vi "AM.vi"() -> ()   [LabVIEW 2017]
uses:
  <vilib>/sound2/lvsound2.llb/Sampling Mode.ctl
  <vilib>/sound2/lvsound2.llb/Sound Data Format.ctl
  <vilib>/Utility/error.llb/DialogType.ctl
  <vilib>/express/express analysis/Spectral/Block/exnSpectralBlock spectral measurements RMS poly.vi
  <vilib>/express/express analysis/Spectral/Block/exnSpectralBlock spectral measurements RMS WFM.vi
  <vilib>/sound2/lvsound2.llb/Sound Output Write (DBL Single).vi
  <vilib>/express/express analysis/Spectral/XNode/ExpressSpectralMeasurementsBlockNode.xnode
panel:
  in  "stop":bool
  out "Ausgang: Zeitbild":dbl[](graph)
  out "Ausgang: Frequenzbild":cluster{"f0":dbl, "df":dbl, "magnitude":dbl[]}(graph)={"f0"=0.0, "df"=2.2675736961451248e-05, "magnitude"=array[22050 elements]}
  in  "Modulationsgrad m":dbl=0.2
  in  "Signalamplitude 2":dbl=3.0
  in  "Signalamplitude 1":dbl=1.0
  in  "Signalfrequenz 2":dbl=1000.0
  in  "Signalfrequenz 1":dbl=700.0
  in  "Trägerfrequenz":dbl=10000.0
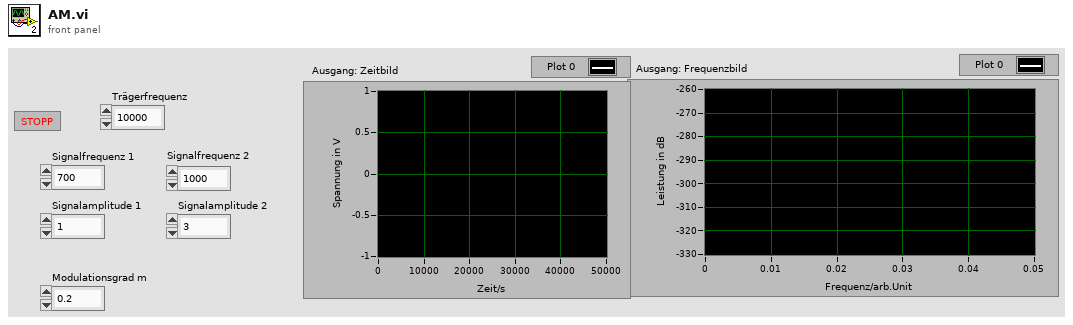
[diagram p1: front panel]
types:
  T1 = typedef "Sound Data Format.ctl" = cluster{"sample rate (S/s)":dbl, "number of channels":i32, "bits per sample":i32}
  T2 = cluster{"averaging mode":u16, "weighting mode":u16, "number of averages":u32}
  T3 = cluster{"dB On (F)":bool, "unwrap phase (F)":bool, "convert to degree (F)":bool}
  T4 = typedef "DialogType.ctl" = u16
  T5 = typedef "Sampling Mode.ctl" = i32
  T6 = typedef "Sound Output Task ID.ctl" = u32
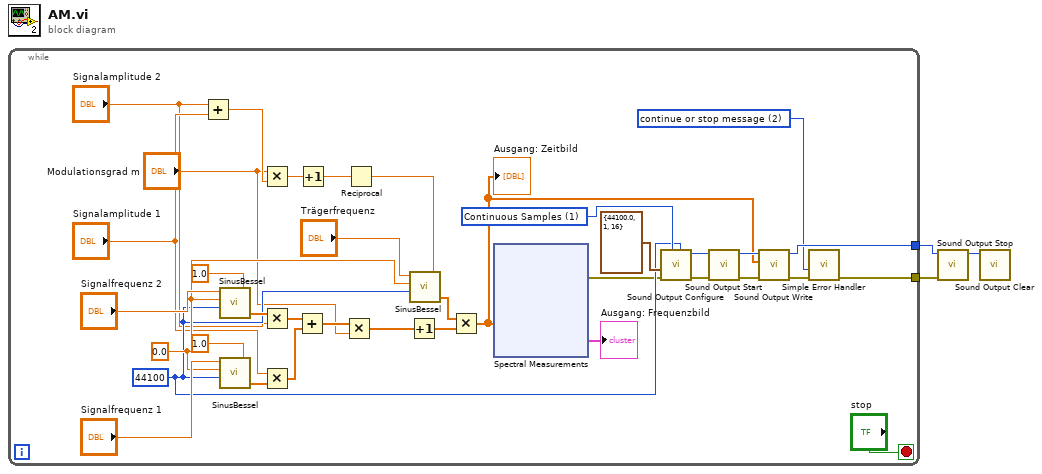
[diagram p0: block diagram]
diagram:
  n1 = while {
    tunnel: [w15] -> w2
    tunnel: [w17] -> w1
    stop <- "stop" stop-if-true
    w14 = T4 2 items=["no dialog", "OK message", "continue or stop message", "OK message + warnings", "continue/stop + warnings"] ("type of dialog (OK msg:1)")
    w13 = 44100 ("number of samples/ch")
    w24 = T5 1 items=["Finite Samples", "Continuous Samples"] ("sample mode")
    w33 = 0.0 ("Phase phi")
    n2 = Add(x="Signalamplitude 2", y="Signalamplitude 1") -> (x+y=w9:dbl)
    n3 = call "SinusBessel.vi"("Amplitude A"=1.0, "Zahl der Punkte N"=w13, "Phase phi"=w33, "Frequenz f"="Signalfrequenz 2") -> ("y"=w37:dbl[])  [unwired: 1 in, 1 out]
    n4 = call "SinusBessel.vi"("Amplitude A"=1.0, "Zahl der Punkte N"=w13, "Phase phi"=w33, "Frequenz f"="Signalfrequenz 1") -> ("y"=w29:dbl[])  [unwired: 1 in, 1 out]
    n5 = Multiply(x="Modulationsgrad m", y=w9) -> (x*y=w7:dbl)
    n6 = Multiply(x=w37, y="Signalamplitude 2") -> (x*y=w25:dbl[])
    n7 = Multiply(x="Signalamplitude 1", y=w29) -> (x*y=w27:dbl[])
    n8 = Add(x=w25, y=w27) -> (x+y=w36:dbl[])
    n9 = Increment(x=w7) -> (x+1=w6:dbl)
    n10 = Multiply(x=w36, y="Modulationsgrad m") -> (x*y=w35:dbl[])
    n11 = Reciprocal(x=w6) -> (1/x=w5:dbl)
    n12 = Increment(x=w35) -> (x+1=w32:dbl[])
    n13 = call "SinusBessel.vi"("Amplitude A"=w5, "Zahl der Punkte N"=w13, "Phase phi"=w33, "Frequenz f"="Trägerfrequenz") -> ("y"=w31:dbl[])  [unwired: 1 in, 1 out]
    n14 = Multiply(x=w31, y=w32) -> (x*y=w18:dbl[])
    "Ausgang: Zeitbild" <- w18
    n15 = xnode "Spectral Measurements"("Signals"=w18) -> ("FFT - (RMS)"=→"Ausgang: Frequenzbild":cluster{"f0":dbl, "df":dbl, "magnitude":dbl[]}, "error out"=w4:errorcluster)  [unwired: 1 in, 1 out]
    n16 = call <vilib>:"Sound Output Configure.vi"("number of samples/ch"=w13, "sample mode"=w24, "error in (no error)"=w4, "sound format"=T1 {"sample rate (S/s)"=44100.0, "number of channels"=1, "bits per sample"=16}) -> ("error out"=w23:errorcluster, "task ID"=w20:T6)  [unwired: 6 in]
    n17 = call <vilib>:"Sound Output Start.vi"("error in (no error)"=w23, "task ID"=w20) -> ("error out"=w22:errorcluster, "task ID out"=w19:T6)  [unwired: 8 in]
    n18 = call-poly <vilib>:"Sound Output Write.vi"("error in (no error)"=w22, "data"=w18, "task ID"=w19) -> ("error out"=w16:errorcluster, "task ID out"=w17:T6)  [unwired: 7 in]
    n19 = call <vilib>:"Simple Error Handler.vi"("type of dialog (OK msg:1)"=w14, "error in (no error)"=w16) -> ("error out"=w15:errorcluster)  [unwired: 3 in, 4 out]
  }
  n20 = call <vilib>:"Sound Output Stop.vi"("error in (no error)"=w2, "task ID"=w1) -> ("task ID out"=w3:T6)  [unwired: 8 in, 1 out]
  n21 = call <vilib>:"Sound Output Clear.vi"("task ID"=w3) -> ()  [unwired: 10 in, 1 out]
